vi "Write id.vi"(8 "error in (no error)":errorcluster, 10 "id":string, 11 "Tool Path in":refnum<class "Tool Path.lvclass">) -> (0 "error out":errorcluster, 3 "Tool Path out":refnum<class "Tool Path.lvclass">)   [LabVIEW 2019, in "Tool Path.lvclass"]
uses:
  Tool Path.lvclass
  Tool Object/Tool Object.lvclass
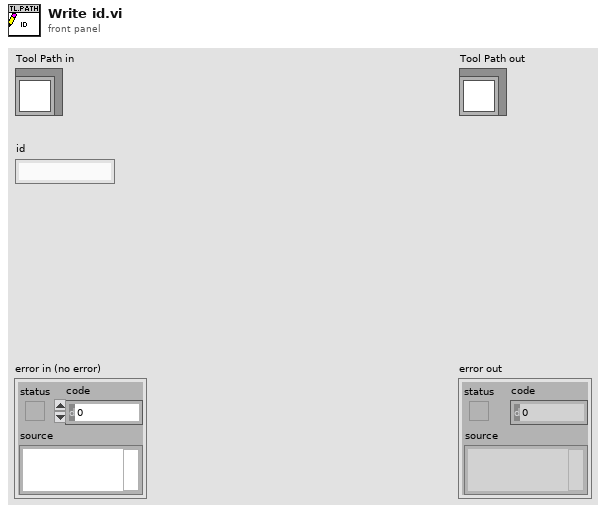
[diagram p1: front panel]
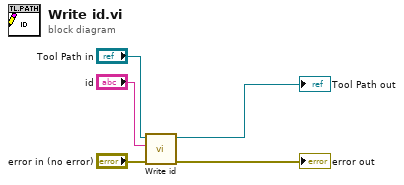
[diagram p0: block diagram]
diagram:
  n1 = call-parent "Write id.vi"("error in (no error)"="error in (no error)", "id"="id", "Tool Object in"="Tool Path in") -> ("error out"=→"error out":errorcluster, "Tool Object out"=→"Tool Path out":refnum<class "Tool Path.lvclass">)  [unwired: 7 in]
